vi "WSS Modes to Word.vi"(11 "Wheel Speed Sensor Modes":T1) -> (3 "Wheel Speed Sensor Word":u16)   [LabVIEW 2014, in "SLSC configuration Shared.lvlib"]
doc: "Converts four faults to a fault word."
uses:
  SLSC configuration Shared.lvlib
  WSS Mode Array.ctl
  WSS Mode.ctl
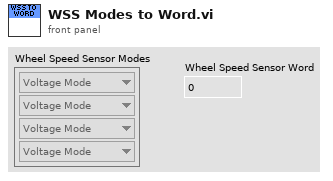
[diagram p1: front panel]
types:
  T1 = typedef "SLSC configuration Shared.lvlib/WSS Mode Array.ctl" = T2[]
  T2 = typedef "SLSC configuration Shared.lvlib/WSS Mode.ctl" = enum8{"Voltage Mode", "Current Mode"}
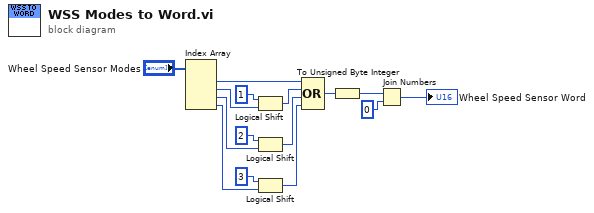
[diagram p0: block diagram]
diagram:
  n1 = Index Array(array="Wheel Speed Sensor Modes") -> (element #1=w12:T2, element #2=w9:T2, element #3=w6:T2, element #4=w4:T2)  [unwired: 4 in]
  n2 = Logical Shift(y=u16 1, x=w9) -> (x << y=w13:u32)
  n3 = Logical Shift(y=u16 2, x=w6) -> (x << y=w14:u32)
  n4 = Logical Shift(y=i16 3, x=w4) -> (x << y=w10:u32)
  n5 = Compound Arithmetic op=OR(w12, w13, w14, w10) -> (w15:u32)
  n6 = To Unsigned Byte Integer(number=w15) -> (unsigned 8bit integer=w3:u8)
  n7 = Join Numbers(hi=w3, lo=u8 0) -> ((hi.lo)=→"Wheel Speed Sensor Word":u16)
